vi "VID_RES_PHS_LMT_CHK.vi"(1 "IF":dbl=1.0, 2 "Resolution":dbl=1.0, 3 "Phase":dbl=180.0, 4 "SampCount":i32=180, 5 "error in":errorcluster) -> (14 "error out":errorcluster, 15 "IF":dbl=1.0, 16 "Resolutiuon":dbl=1.0, 17 "Phase":dbl, 18 "SampCount":i32)   [LabVIEW 2018, in "PNA-X.lvlib"]
uses:
  PNA-X.lvlib
panel:
  in  "Limits":T1={"IFMax"=1000000.0, "IFMin"=1.0, "ResMax"=10000000.0, "ResMin"=1.0, "PhsMax"=360.0, "PhsMin"=-360.0, "CountMax"=360, "CountMin"=-360}
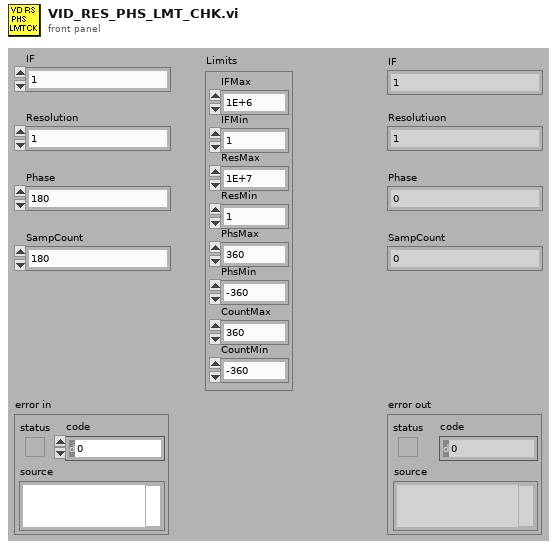
[diagram p1: front panel]
types:
  T1 = cluster{"IFMax":dbl, "IFMin":dbl, "ResMax":dbl, "ResMin":dbl, "PhsMax":dbl, "PhsMin":dbl, "CountMax":i32, "CountMin":i32}
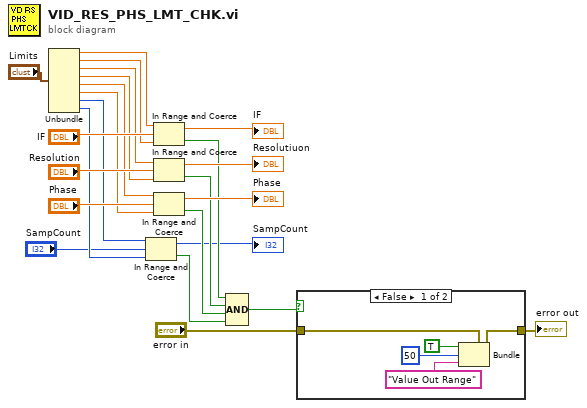
[diagram p0: block diagram]
diagram:
  n1 = Unbundle("Limits") -> ("IFMax"=w11:dbl, "IFMin"=w12:dbl, "ResMax"=w13:dbl, "ResMin"=w14:dbl, "PhsMax"=w15:dbl, "PhsMin"=w16:dbl, "CountMax"=w4:i32, "CountMin"=w3:i32)
  n2 = In Range and Coerce(upper limit=w4, x="SampCount", lower limit=w3) -> (coerced(x)=→"SampCount":i32, In Range?=w5:bool)
  n3 = In Range and Coerce(upper limit=w11, x="IF", lower limit=w12) -> (coerced(x)=→"IF":dbl, In Range?=w10:bool)
  n4 = In Range and Coerce(upper limit=w13, x="Resolution", lower limit=w14) -> (coerced(x)=→"Resolutiuon":dbl, In Range?=w9:bool)
  n5 = In Range and Coerce(upper limit=w15, x="Phase", lower limit=w16) -> (coerced(x)=→"Phase":dbl, In Range?=w8:bool)
  n6 = Compound Arithmetic op=AND(w10, w9, w8, w5) -> (w7:bool)
  n7 = case shown="False" w7 {
    tunnel: "error in" -> [w28 w30]
    tunnel: [w29 w30] -> w24
    frame False {
      n8 = Bundle(cluster=w28, "status"=TRUE, "code"=50, "source"="Value Out Range") -> (w29:errorcluster)
    }
    frame True {
    }
  }
  "error out" <- w24
